vi "Configure Instrument Mode.vi"(0 "VISA resource name":refnum<visa-resource-name>, 1 "Unit Address (1)":u8=1 min=1 max=254, 5 "Instrument Mode (0: Normal)":u8(ring) items=["Normal", "StandBy", "Configuration"], 11 "error in (no error)":errorcluster) -> (4 "VISA resource name out":refnum<visa-resource-name>, 15 "error out":errorcluster)   [LabVIEW 2010, in "Eurotherm 32xx Series.lvlib"]
doc: "This VI sets instrument mode.\n\nWarning: Changing default value interrupts working process (device will not control).\nIt is recommended that the device be disconnected from any active process."
uses:
  <instrlib>/Eurotherm 32xx Series/Eurotherm 32xx Series.lvlib
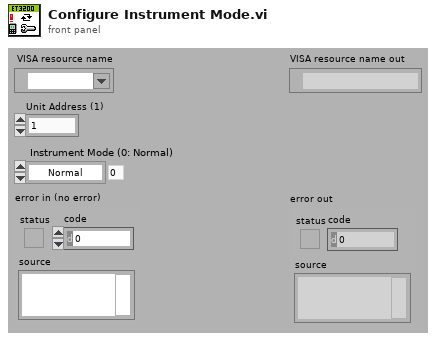
[diagram p1: front panel]
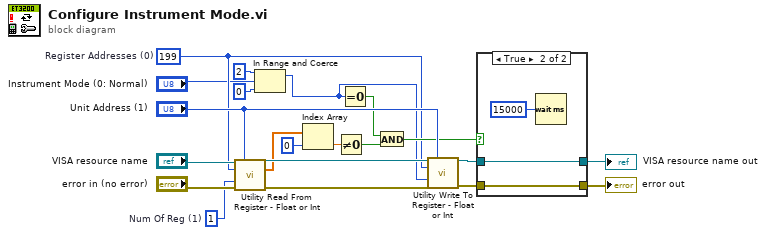
[diagram p0: block diagram]
diagram:
  w16 = u16 1  # Num Of Reg (1)
  w5 = u16 199  # Register Addresses (0)
  n1 = call <instrlib>:"Utility Read From Register - Float or Int.vi"("VISA resource name"="VISA resource name", "Unit Address (1)"="Unit Address (1)", "Register Address (0)"=w5, "Num Of Reg (1)"=w16, "error in (no error)"="error in (no error)") -> ("VISA resource name out"=w19:refnum<visa-resource-name>, "Data"=w15:sgl[], "error out"=w20:errorcluster)  [unwired: 8 in]
  n2 = In Range and Coerce(upper limit=u8 2, x="Instrument Mode (0: Normal)", lower limit=u8 0) -> (coerced(x)=w3:u8)  [unwired: 1 out]
  n3 = Index Array(array=w15, index=0) -> (element=w13:sgl)
  n4 = Not Equal To 0?(x=w13) -> (x != 0?=w12:bool)
  n5 = Equal To 0?(x=w3) -> (x = 0?=w11:bool)
  n6 = And(x=w11, y=w12) -> (x .and. y?=w6:bool)
  n7 = call <instrlib>:"Utility Write To Register - Float or Int.vi"("VISA resource name"=w19, "Unit Address (1)"="Unit Address (1)", "Register Address (0)"=w5, "Data (0)"=w3, "error in (no error)"=w20) -> ("VISA resource name out"=w10:refnum<visa-resource-name>, "error out"=w8:errorcluster)  [unwired: 9 in]
  n8 = case shown="True" w6 {
    tunnel: w10 -> [w23 w26]
    tunnel: [w23 w26] -> w9
    tunnel: w8 -> [w22 w25]
    tunnel: [w22 w25] -> w7
    frame False {
    }
    frame True {
      n9 = Wait (ms)(milliseconds to wait=u32 15000) -> ()  [unwired: 1 out]
    }
  }
  "error out" <- w7
  "VISA resource name out" <- w9
